vi "Set translation speed.vi"(8 "error in (no error)":errorcluster, 11 "ImageStack in":refnum<class "ImageStack.lvclass">) -> (0 "error out":errorcluster, 3 "ImageStack out":refnum<class "ImageStack.lvclass">)   [LabVIEW 2012, in "ImageStack.lvclass"]
uses:
  ImageStack.lvclass
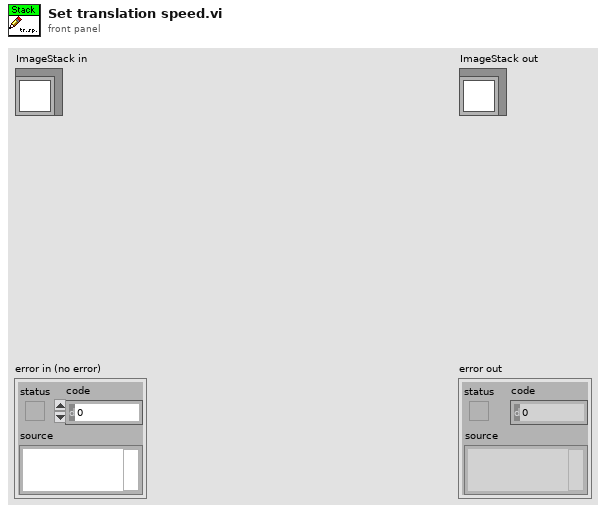
[diagram p1: front panel]
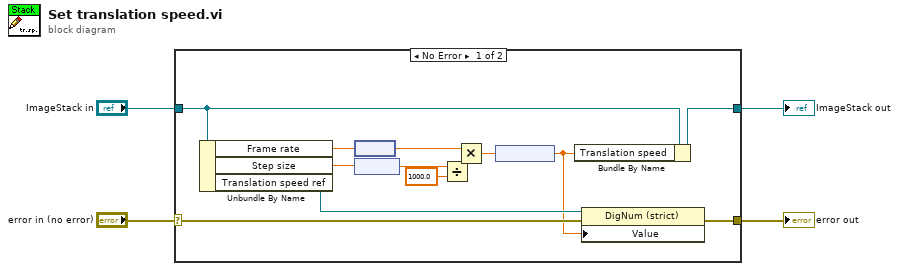
[diagram p0: block diagram]
diagram:
  n1 = case shown="No Error" "error in (no error)" {
    selector: "error in (no error)" -> [w7 w19]
    tunnel: [w6 w19] -> w3
    tunnel: [w11 w18] -> w1
    tunnel: "ImageStack in" -> [w12 w18]
    frame No Error {
      n2 = Unbundle By Name(w12) -> ("Frame rate"=w10:dbl[unit], "Step size"=w9:dbl[unit], "Translation speed ref"=w8:refnum<vi>)
      n3 = node(w10) -> (w16:dbl)
      n4 = node(w9) -> (w17:dbl)
      n5 = Divide(x=w17, y=1000.0) -> (x/y=w15:dbl)
      n6 = Multiply(x=w16, y=w15) -> (x*y=w13:dbl)
      n7 = node(w13) -> (w5:dbl[unit])
      n8 = Bundle By Name(cluster=w12, "Translation speed"=w5) -> (w11:refnum<class "ImageStack.lvclass">)
      n9 = property class="DigNum (strict)"(reference=w8, error in=w7, "Value"=w5) -> (error out=w6:errorcluster)  [unwired: 1 out]
    }
    frame Error {
    }
  }
  "error out" <- w3
  "ImageStack out" <- w1
